vi "Set Current Record from Keypad.vi"(8 "error in (no error)":errorcluster, 10 "Keypad":T1, 11 "ATM Controller in":refnum<class "ATM Controller.lvclass">) -> (0 "error out":errorcluster, 3 "ATM Controller out":refnum<class "ATM Controller.lvclass">)   [LabVIEW 2019, in "ATM Controller.lvlib" / "ATM Controller.lvclass"]
uses:
  ATM Controller.lvclass
  Simulated User Console Actor/Simulated User Console Actor/Keypad - Cluster.ctl
  Simulated User Console Actor/Simulated User Console Actor/Simulated User Console Actor.lvclass
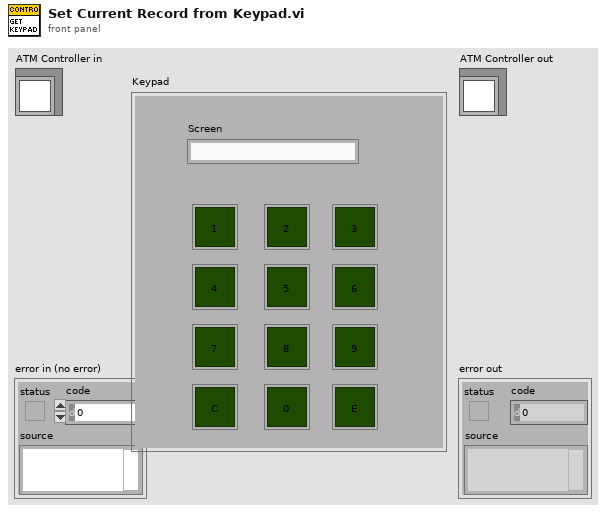
[diagram p1: front panel]
types:
  T1 = typedef "Simulated User Console Actor.lvlib/Simulated User Console Actor.lvclass/Keypad - Cluster.ctl" = cluster{"1":bool, "1 2":bool, "1 3":bool, "1 4":bool, "1 5":bool, "1 6":bool, "1 7":bool, "1 8":bool, "1 9":bool, "C":bool, "1 11":bool, "E":bool, "Screen":string}
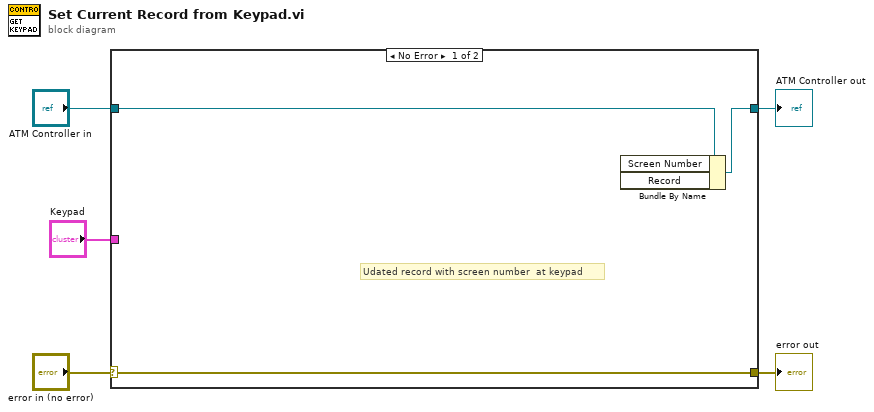
[diagram p0: block diagram]
diagram:
  n1 = case shown="No Error" "error in (no error)" {
    selector: "error in (no error)" -> [w8 w10]
    tunnel: [w8 w10] -> w4
    tunnel: [w7 w9] -> w2
    tunnel: "ATM Controller in" -> [w6 w9]
    tunnel: "Keypad" -> [_ _]
    frame No Error {
      # "Udated record with screen number  at keypad"
      n2 = Bundle By Name(cluster=w6) -> (w7:refnum<class "ATM Controller.lvclass">)  [unwired: 2 in]
    }
    frame Error {
    }
  }
  "error out" <- w4
  "ATM Controller out" <- w2
